vi "IC_SnapAndSaveBMP.vi"(1 "Filename":string, 2 "ICImagingControl 3":refnum<k7>) -> (0 "ICImagingControl 2":refnum<k7>)   [LabVIEW 2020]
doc: "This VI calls MemorySnapImage and saves the snaped image as bitmap file."
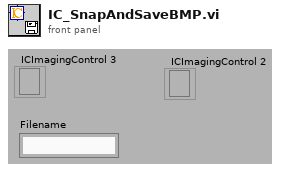
[diagram p1: front panel]
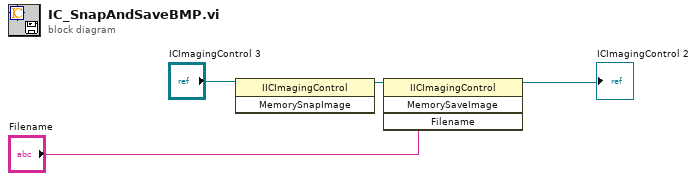
[diagram p0: block diagram]
diagram:
  n1 = invoke class="IICImagingControl" method="MemorySnapImage"(reference="ICImagingControl 3") -> (reference out=w2:refnum<k7>)  [unwired: 2 in, 2 out]
  n2 = invoke class="IICImagingControl" method="MemorySaveImage"(reference=w2, "Filename"="Filename") -> (reference out=→"ICImagingControl 2":refnum<k7>)  [unwired: 2 in, 3 out]
